vi "Joystick gerakan.vi"() -> ()   [LabVIEW 2019]
uses:
  <vilib>/Platform/TimedLoop/XDataNode/wakeup.ctl
  <vilib>/Platform/TimedLoop/XDataNode/XDNodeRunTimeDep.lvlib
  <vilib>/Platform/TimedLoop/XDataNode/nitl_modes.ctl
  <vilib>/Platform/TimedLoop/XDataNode/timing_clust.ctl
  <vilib>/platform/TimedLoop/XDataNode/XDataNode.xnode
  <vilib>/rvi/interface/nirviReadWriteControl/nirviReadWriteControl.xnode
  <vilib>/rvi/interface/Simulation/niFpgaSimulationCallBeginRW.vi
  <vilib>/rvi/errors/niLvFpgaAdjustHostInterfaceError.vi
  <vilib>/robotics/Steering/Steering Frame/NI_Robotics_Steering Frame.lvclass
  <vilib>/robotics/Steering/Mecanum Steering Frame/NI_Robotics_Mecanum Steering Frame.lvclass
  <vilib>/robotics/Steering/Class Type Definitions/Mecanum Steering Frame.ctl
  <vilib>/robotics/Steering/Class Type Definitions/NI_Robotics_Steering Class Types.lvlib
  <vilib>/robotics/Steering/Mecanum Wheel/Roller Orientation.ctl
  <vilib>/robotics/Steering/Mecanum Wheel/NI_Robotics_Mecanum Wheel.lvclass
  <vilib>/robotics/Steering/Wheel/Rotation Direction.ctl
  <vilib>/robotics/Steering/Wheel/NI_Robotics_Wheel.lvclass
  <vilib>/robotics/Steering/Wheel/Wheel Parameters.ctl
  <vilib>/robotics/Steering/Mecanum Steering Frame/Create Mecanum Steering Frame.vi
  <vilib>/robotics/Steering/Mecanum Wheel/Create Mecanum Wheel.vi
  <vilib>/robotics/Steering/Create Steering Frame/NI_Robotics_Create Steering Frame.xnode
  <vilib>/rvi/interface/nirviCloseFPGA/nirviCloseFPGA.xnode
  <vilib>/rvi/interface/nirviOpenFPGA/nirviOpenFPGA.xnode
  <vilib>/Utility/error.llb/Error Cluster From Error Code.vi
  <vilib>/FPGAPlugInAG/Dynamic/niLvFpga_Close_Dynamic.vi
  Collin's Project/FPGA Bitfiles/MRmecanum_FPGATarget_FPGAMainModified_TerasRobot_LKSN2021.lvbitx
  <vilib>/vision/NI_Vision_Development_Module.lvlib
  NiFpgaLv.dll
  <vilib>/robotics/Steering/Steering Frame/Apply Steering Frame Velocity to Motors.vi
  C:/Program Files (x86)/National Instruments/LabVIEW 2019/vi.lib/robotics/Steering/Special Steering Frame/NI_Robotics_Special Steering Frame.lvclass
  C:/Program Files (x86)/National Instruments/LabVIEW 2019/vi.lib/robotics/Steering/Steering Frame/NI_Robotics_Steering Frame.lvclass
  <vilib>/FPGAPlugInAG/myRIO-1900/niLvFpga_Open_myRIO-1900.vi
  <vilib>/rvi/interface/common/dynamic/niFpgaDynamicAddResources.vi
panel:
  out "Flashlight Number":dbl
  in  "Servo 2":u16=1950
  in  "Max.Servo 2":u16=5000
  in  "Min.Servo 2":u16=1500
  in  "Step Servo 2":u16=50
  out "Kanan Depan":bool
  out "Kanan Belakang":bool
  out "Belakang Kanan":bool
  out "Belakang Kiri":bool
  out "Kiri Belakang":bool
  in  "Stop":bool
  out "Image Out":T1(plugin-control)
  out "Kiri Depan":bool
  out "Depan":bool
  in  "Max.Servo 3":u16=5000
  in  "Min.Servo 3":u16=4400
  in  "Max. Kcp":dbl=500.0
  in  "Min. Kcp":dbl=500.0
  in  "Step Servo 3":u16=50
  in  "Servo 3":u16=5000
  in  "Motor 5":i16=2500
  in  "Putaran":dbl=1700.0
  in  "Kecepatan":dbl=500.0
  # "Maju\nMundur\nKiri\nKanan"
  # "Default Value\n2500"
  # "Putar Kiri\nPutar Kanan"
  # "Std Value : 815"
  # "Std Value : 300\nMin Value : 150\nMax. Value : 400"
  # "Default Value"
  # "Default 3000"
  # "Default 3500"
  # "Default 50"
  # "Servo 3\nDefault Value\n1500"
  # "Default 1000"
  # "Default 2000"
  # "Default 50"
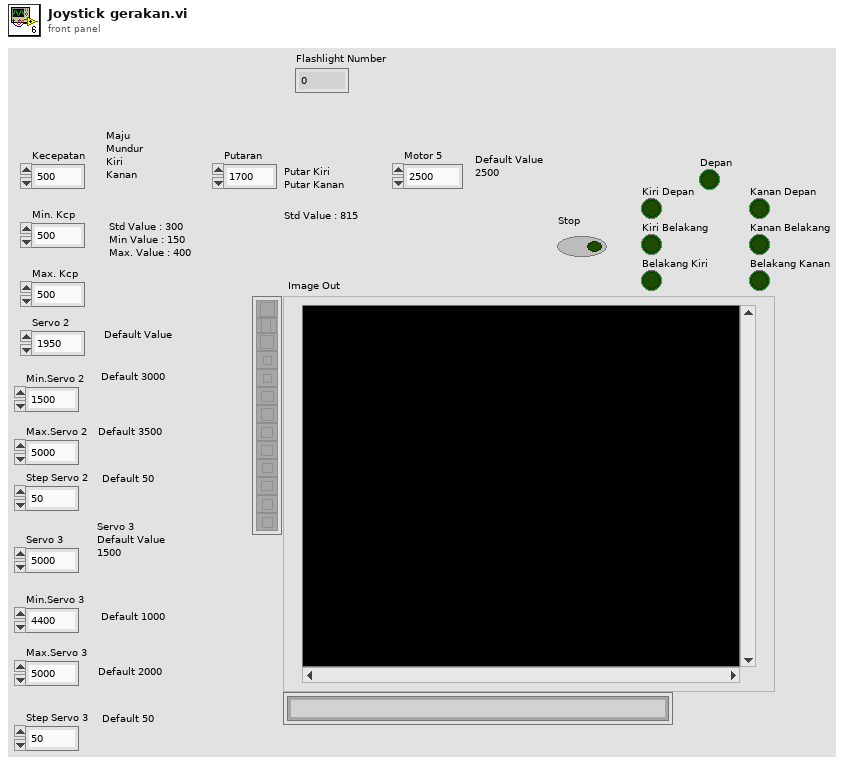
[diagram p1: front panel]
types:
  T1 = typedef "IMAQ Image.ctl" = refnum<image>
  T2 = typedef "NI_Robotics_Steering Class Types.lvlib/Mecanum Steering Frame.ctl" = refnum<class "NI_Robotics_Mecanum Steering Frame.lvclass">
  T3 = typedef "XDNodeRunTimeDep.lvlib/timing_clust.ctl" = cluster{"Expected End [f-1]":u64, "Actual End [f-1]":u64, "Finished Late? [f-1]":bool, "Expected End [i-1]":u64, "Actual End [i-1]":u64, "Finished Late? [i-1]":bool, "Expected Start [i]":u64, "Actual Start [i]":u64, "Expected Start [f]":u64, "Actual Start [f]":u64, "Source Name":string, "Structure Name":string, "Period":i64, "Deadline":i64, "Offset":i64, "Start":i64, "Priority":i32, "Timeout":i32, "Mode":T4, "Wakeup Reason":T5, "Error":errorcluster, "Source Type":string, "Secondary Source Type":string, "Global End Time":u64, "Global Start Time":u64, "Frame Duration":u64, "Iteration Duration":u64, "Assigned CPU":i32, "I/O Scan Engine Mode":u32}
  T4 = typedef "XDNodeRunTimeDep.lvlib/nitl_modes.ctl" = enum32{"No Change", "Process missed periods, maintain original phase", "Discard missed periods, maintain original phase", "Process missed periods, ignore original phase", "Discard missed periods, ignore original phase"}
  T5 = typedef "XDNodeRunTimeDep.lvlib/wakeup.ctl" = enum32{"Normal", "Aborted", "Asynchronous wakeup", "Timing source error", "Timed loop error", "Timeout"}
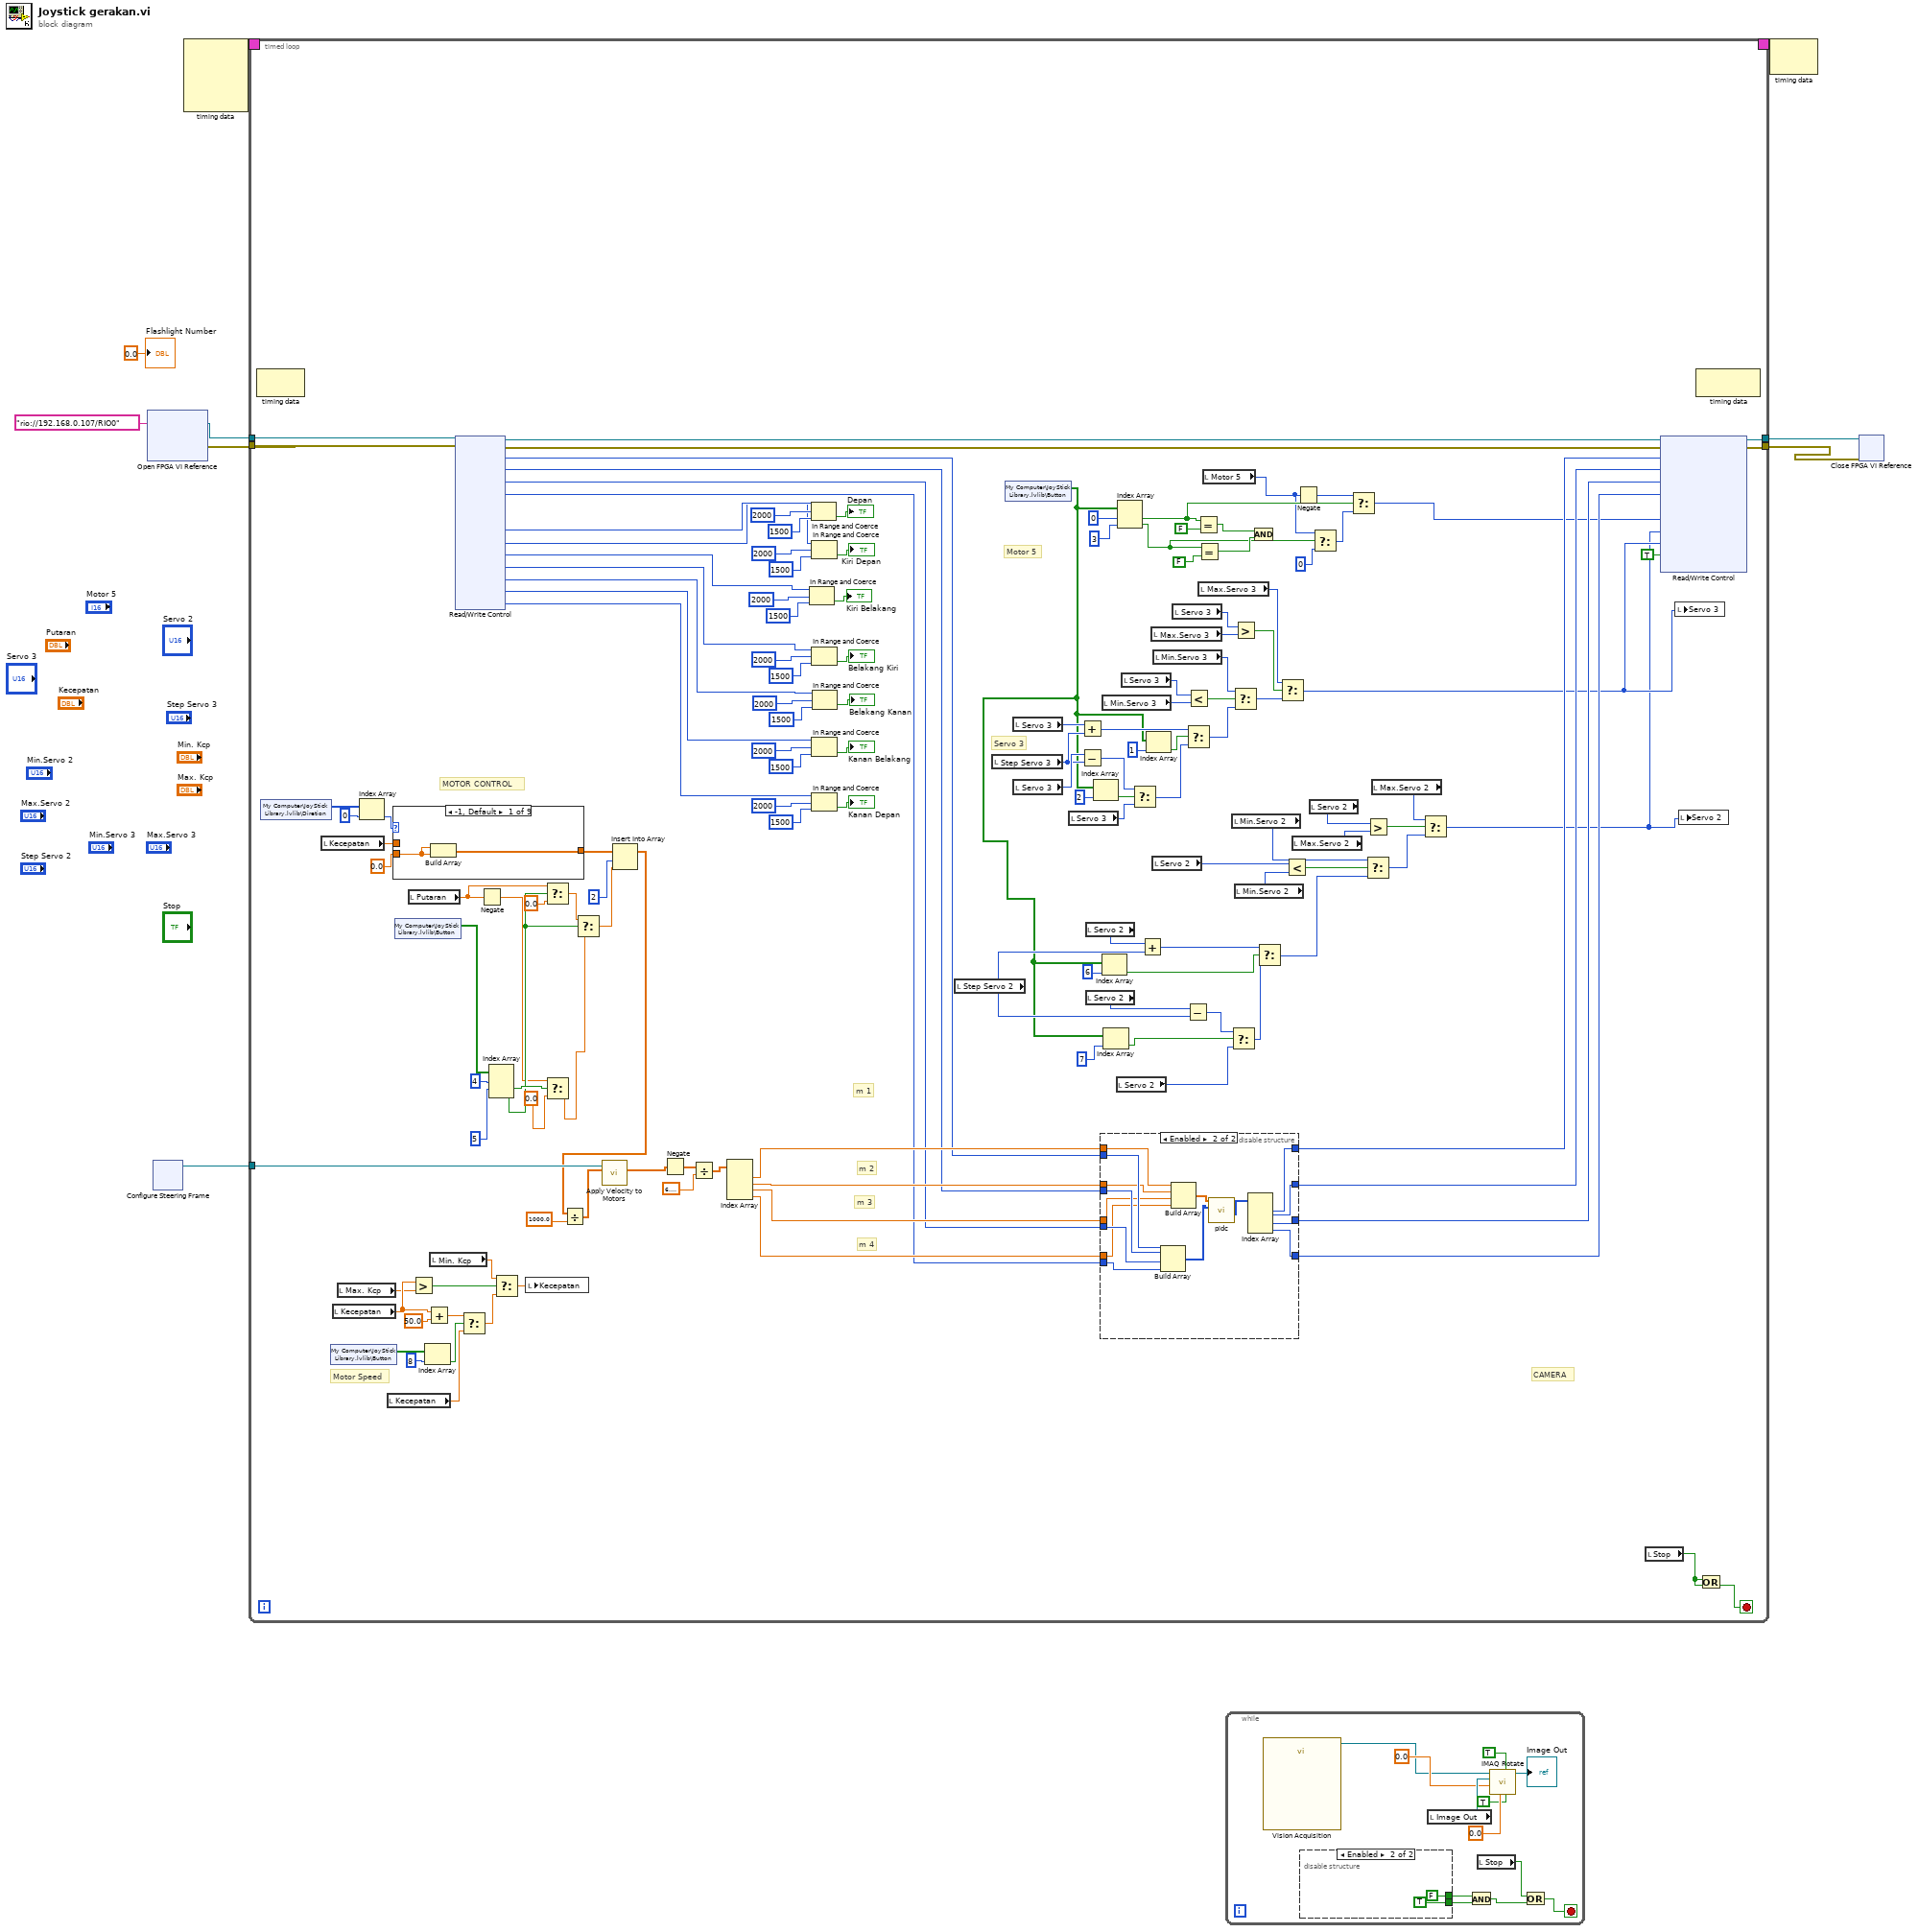
[diagram p0: block diagram]
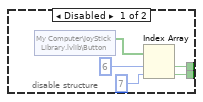
[diagram p2: hidden frame]
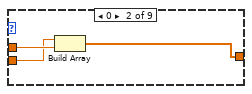
[diagram p3: hidden frame]
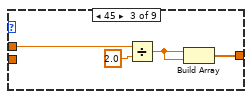
[diagram p4: hidden frame]
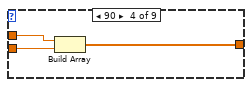
[diagram p5: hidden frame]
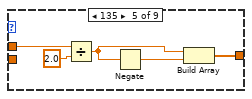
[diagram p6: hidden frame]
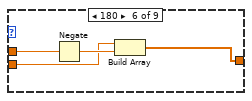
[diagram p7: hidden frame]
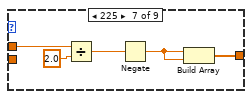
[diagram p8: hidden frame]
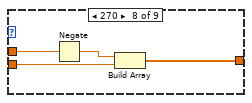
[diagram p9: hidden frame]
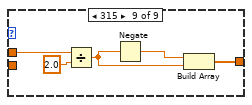
[diagram p10: hidden frame]
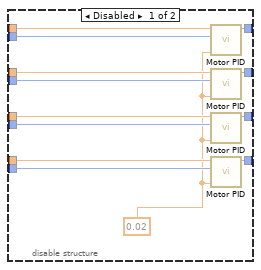
[diagram p11: hidden frame]
diagram:
  n1 = xnode "Open FPGA VI Reference"("resource name"=tag "rio://192.168.0.107/RIO0") -> ("FPGA VI Reference Out"=w4:refnum<k20>, "error out"=w3:errorcluster)  [unwired: 1 in]
  n2 = xnode ("Configure Steering Frame")() -> ("mecanum steering frame out"=w7:T2)  [unwired: 1 in, 1 out]
  n3 = node-c288() -> (w9:T3)  [unwired: 4 in]
  n4 = timed-loop {
    timing: w9 -> [_]
    timing-out: [_] -> w8
    tunnel: w4 -> [w23]
    tunnel: w3 -> [w153]
    tunnel: [w155] -> w6
    tunnel: [w154] -> w5
    tunnel: w7 -> [w152]
    stop <- w71 stop-if-true
    # "CAMERA"
    # "Motor Speed"
    # "Servo 3"
    # "Motor 5"
    # "MOTOR CONTROL"
    # "m 4"
    # "m 3"
    # "m 2"
    # "m 1"
    n5 = node-c288() -> ()  [unwired: 1 in, 1 out]
    n6 = shared-variable "My Computer\\JoyStick Library.lvlib\\Diretion"() -> (w133:i32[])  [unwired: 1 in, 1 out]
    n7 = local read "Kecepatan"() -> (w117:dbl)
    n8 = shared-variable "My Computer\\JoyStick Library.lvlib\\Button"() -> (w100:bool[])  [unwired: 1 in, 1 out]
    n9 = local read "Kecepatan"() -> (w94:dbl)
    n10 = local read "Max. Kcp"() -> (w89:dbl)
    n11 = Index Array(array=w133, index=0) -> (element=w131:i32)
    n12 = local read "Kecepatan"() -> (w91:dbl)
    n13 = case shown="-1, Default" w131 {
      tunnel: [w156 w160 w164 w165 w172 w176 w181 w182 w189] -> w127
      tunnel: w117 -> [_ w159 w162 w167 w170 w175 w180 w185 w186]
      tunnel: 0.0 ("element") -> [w157 w158 _ w166 _ w173 _ w183 _]
      frame -1, Default {
        n14 = Build Array(w157, w157) -> (w156:dbl[])
      }
      frame 0 {
        n15 = Build Array(w158, w159) -> (w160:dbl[])
      }
      frame 45 {
        n16 = Divide(x=w162, y=2.0) -> (x/y=w163:dbl)
        n17 = Build Array(w163, w163) -> (w164:dbl[])
      }
      frame 90 {
        n18 = Build Array(w167, w166) -> (w165:dbl[])
      }
      frame 135 {
        n19 = Divide(x=w170, y=2.0) -> (x/y=w169:dbl)
        n20 = Negate(x=w169) -> (-x=w171:dbl)
        n21 = Build Array(w169, w171) -> (w172:dbl[])
      }
      frame 180 {
        n22 = Negate(x=w175) -> (-x=w174:dbl)
        n23 = Build Array(w173, w174) -> (w176:dbl[])
      }
      frame 225 {
        n24 = Divide(x=w180, y=2.0) -> (x/y=w178:dbl)
        n25 = Negate(x=w178) -> (-x=w179:dbl)
        n26 = Build Array(w179, w179) -> (w181:dbl[])
      }
      frame 270 {
        n27 = Negate(x=w185) -> (-x=w184:dbl)
        n28 = Build Array(w184, w183) -> (w182:dbl[])
      }
      frame 315 {
        n29 = Divide(x=w186, y=2.0 ("Kecepatan")) -> (x/y=w187:dbl)
        n30 = Negate(x=w187) -> (-x=w190:dbl)
        n31 = Build Array(w190, w187) -> (w189:dbl[])
      }
    }
    n32 = shared-variable "My Computer\\JoyStick Library.lvlib\\Button"() -> (w130:bool[])  [unwired: 1 in, 1 out]
    n33 = local read "Putaran"() -> (w115:dbl)
    n34 = Greater?(x=w94, y=w89) -> (0:w98:bool)
    n35 = Index Array(array=w100, index=8) -> (element=w96:bool)
    n36 = Add(x=w94, y=50.0) -> (x+y=w95:dbl)
    n37 = local read "Min. Kcp"() -> (w97:dbl)
    n38 = xnode "Read/Write Control"("FPGA VI Reference In"=w23, "error in"=w153) -> ("FPGA VI Reference Out"=w77:refnum<k20>, "error out"=w72:errorcluster, "ENC M1"=w145:i32, "ENC M2"=w144:i32, "ENC M3"=w143:i32, "ENC M4"=w142:i32, "IR 1"=w76:u16, "IR 3"=w67:u16, "IR 4"=w54:u16, "IR 5"=w53:u16, "IR 6"=w52:u16, "IR 7"=w51:u16, "IR 8"=w47:u16)  [unwired: 2 out]
    n39 = Select(t=w95, s=w96, f=w91) -> (s? t:f=w92:dbl)
    n40 = Negate(x=w115) -> (-x=w114:dbl)
    n41 = Index Array(array=w130, index #1=4 ("index"), index #2=5 ("index")) -> (element #1=w119:bool, element #2=w122:bool)  [unwired: 1 in, 1 out]
    n42 = Select(t=w97, s=w98, f=w92) -> (s? t:f=w90:dbl)
    n43 = local write "Kecepatan"(w90) -> ()
    n44 = Select(t=w115, s=w119, f=0.0) -> (s? t:f=w120:dbl)
    n45 = Select(t=w114, s=w122, f=0.0) -> (s? t:f=w121:dbl)
    n46 = Select(t=w120, s=w119, f=w121) -> (s? t:f=w118:dbl)
    n47 = Insert Into Array(array=w127, index=2, new element=w118) -> (w125:dbl[])
    n48 = Divide(x=w125, y=1000.0) -> (x/y=w136:dbl[])
    n49 = call-poly <vilib>:"Apply Velocity to Motors.vi"("steering frame velocity"=w136, "steering frame in"=w152) -> ("ccw motor velocity setpoints"=w150:dbl[])  [unwired: 5 in, 4 out]
    n50 = Negate(x=w150) -> (-x=w151:dbl[])
    n51 = Divide(x=w151, y=6.283185307179586) -> (x/y=w135:dbl[])
    n52 = Index Array(array=w135) -> (element #1=w149:dbl, element #2=w148:dbl, element #3=w147:dbl, element #4=w146:dbl)  [unwired: 4 in]
    n53 = In Range and Coerce(upper limit=w54, x=u16 2000, lower limit=u16 1500 ("y")) -> (In Range?=→"Kiri Belakang":bool)  [unwired: 1 out]
    n54 = In Range and Coerce(upper limit=w76, x=u16 2000, lower limit=u16 1500 ("y")) -> (In Range?=→"Depan":bool)  [unwired: 1 out]
    n55 = In Range and Coerce(upper limit=w67, x=u16 2000, lower limit=u16 1500 ("y")) -> (In Range?=→"Kiri Depan":bool)  [unwired: 1 out]
    n56 = In Range and Coerce(upper limit=w53, x=u16 2000, lower limit=u16 1500 ("y")) -> (In Range?=→"Belakang Kiri":bool)  [unwired: 1 out]
    n57 = In Range and Coerce(upper limit=w51, x=u16 2000, lower limit=u16 1500 ("y")) -> (In Range?=→"Kanan Belakang":bool)  [unwired: 1 out]
    n58 = In Range and Coerce(upper limit=w47, x=u16 2000, lower limit=u16 1500 ("y")) -> (In Range?=→"Kanan Depan":bool)  [unwired: 1 out]
    n59 = In Range and Coerce(upper limit=w52, x=u16 2000, lower limit=u16 1500 ("y")) -> (In Range?=→"Belakang Kanan":bool)  [unwired: 1 out]
    n60 = local read "Step Servo 2"() -> (w41:u16)
    n61 = local read "Step Servo 3"() -> (w101:u16)
    n62 = shared-variable "My Computer\\JoyStick Library.lvlib\\Button"() -> (w11:bool[])  [unwired: 1 in, 1 out]
    n63 = local read "Servo 3"() -> (w110:u16)
    n64 = local read "Servo 3"() -> (w105:u16)
    n65 = local read "Servo 3"() -> (w103:u16)
    n66 = Add(x=w110, y=w101) -> (x+y=w109:u16)
    n67 = Subtract(x=w105, y=w101) -> (x-y=w107:u16)
    n68 = local read "Servo 2"() -> (w43:u16)
    n69 = local read "Servo 2"() -> (w42:u16)
    n70 = Index Array(array=w11, index=2) -> (element=w108:bool)
    n71 = disable-structure shown="Enabled" {
      disable-tunnel: w149 -> [w203 w211]
      disable-tunnel: w148 -> [w202 w212]
      disable-tunnel: w147 -> [w201 w213]
      disable-tunnel: w146 -> [w200 w214]
      disable-tunnel: w145 -> [w199 w215]
      disable-tunnel: w144 -> [w198 w216]
      disable-tunnel: w143 -> [w197 w217]
      disable-tunnel: w142 -> [w196 w218]
      disable-tunnel: [w195 w208] -> w141
      disable-tunnel: [w194 w204] -> w140
      disable-tunnel: [w193 w207] -> w139
      disable-tunnel: [w192 w206] -> w138
      frame Disabled {
        w191 = 0.02
        n72 = call "Motor PID.vi"("dt[s]"=w191, "encoder"=w199, "vel ref[rps]"=w203) -> ("duty cycle"=w195:i16)  [unwired: 6 in, 2 out]
        n73 = call "Motor PID.vi"("dt[s]"=w191, "encoder"=w198, "vel ref[rps]"=w202) -> ("duty cycle"=w194:i16)  [unwired: 6 in, 2 out]
        n74 = call "Motor PID.vi"("dt[s]"=w191, "encoder"=w197, "vel ref[rps]"=w201) -> ("duty cycle"=w193:i16)  [unwired: 6 in, 2 out]
        n75 = call "Motor PID.vi"("dt[s]"=w191, "encoder"=w196, "vel ref[rps]"=w200) -> ("duty cycle"=w192:i16)  [unwired: 6 in, 2 out]
      }
      frame Enabled {
        n76 = Build Array(w215, w216, w217, w218) -> (w209:i32[])
        n77 = Build Array(w211, w212, w213, w214) -> (w210:dbl[])
        n78 = call "pidc.vi"("input encoder 2"=w209, "input rps"=w210) -> ("Output duty cycle"=w205:i16[])  [unwired: 9 in]
        n79 = Index Array(array=w205) -> (element #1=w208:i16, element #2=w204:i16, element #3=w207:i16, element #4=w206:i16)  [unwired: 4 in]
      }
    }
    n80 = local read "Min.Servo 3"() -> (w82:u16)
    n81 = Index Array(array=w11, index=6) -> (element=w44:bool)
    n82 = Index Array(array=w11, index=7) -> (element=w27:bool)
    n83 = local read "Servo 2"() -> (w30:u16)
    n84 = Index Array(array=w11, index #1=0 ("index"), index #2=3 ("index")) -> (element #1=w18:bool, element #2=w16:bool)
    n85 = local read "Servo 3"() -> (w83:u16)
    n86 = Select(t=w107, s=w108, f=w103) -> (s? t:f=w106:u16)
    n87 = Add(x=w43, y=w41) -> (x+y=w28:u16)
    n88 = Index Array(array=w11, index=1) -> (element=w111:bool)
    n89 = local read "Max.Servo 3"() -> (w87:u16)
    n90 = local read "Servo 2"() -> (w26:u16)
    n91 = local read "Min.Servo 3"() -> (w80:u16)
    n92 = local read "Servo 3"() -> (w88:u16)
    n93 = Subtract(x=w42, y=w41) -> (x-y=w31:u16)
    n94 = Less?(x=w83, y=w82) -> (x < y?=w81:bool)
    n95 = Select(t=w109, s=w111, f=w106) -> (s? t:f=w79:u16)
    n96 = Equal?(x=w18, y=FALSE) -> (x = y?=w20:bool)
    n97 = Equal?(x=w16, y=FALSE) -> (x = y?=w19:bool)
    n98 = local read "Max.Servo 3"() -> (w85:u16)
    n99 = local read "Motor 5"() -> (w15:i16)
    n100 = Select(t=w31, s=w27, f=w30) -> (s? t:f=w29:u16)
    n101 = local read "Min.Servo 2"() -> (w36:u16)
    n102 = Greater?(x=w88, y=w87) -> (0:w86:bool)
    n103 = Select(t=w80, s=w81, f=w79) -> (s? t:f=w78:u16)
    n104 = local read "Min.Servo 2"() -> (w40:u16)
    n105 = And(x=w20, y=w19) -> ()  [unwired: 1 out]
    n106 = Select(t=w28, s=w44, f=w29) -> (s? t:f=w24:u16)
    n107 = Select(t=w85, s=w86, f=w78) -> (s? t:f=w84:u16)
    n108 = Less?(x=w26, y=w40) -> (x < y?=w37:bool)
    n109 = local read "Max.Servo 2"() -> (w38:u16)
    n110 = Negate(x=w15) -> (-x=w17:i16)
    n111 = local read "Servo 2"() -> (w39:u16)
    n112 = Select(t=w15, s=w16, f=i16 0) -> (s? t:f=w13:i16)
    n113 = Select(t=w17, s=w18, f=w13) -> (s? t:f=w12:i16)
    n114 = Select(t=w36, s=w37, f=w24) -> (s? t:f=w34:u16)
    n115 = Greater?(x=w39, y=w38) -> (0:w35:bool)
    n116 = local read "Max.Servo 2"() -> (w33:u16)
    n117 = Select(t=w33, s=w35, f=w34) -> (s? t:f=w32:u16)
    n118 = local read "Stop"() -> (w25:bool)
    n119 = xnode "Read/Write Control"("FPGA VI Reference In"=w77, "error in"=w72, "M1"=w141, "M2"=w140, "M3"=w139, "M4"=w138, "M5"=w12, "SERVO 2"=w32, "SERVO 3"=w84, "DIO.A_13.VAL"=TRUE) -> ("FPGA VI Reference Out"=w155:refnum<k20>, "error out"=w154:errorcluster)  [unwired: 2 in]
    n120 = local write "Servo 3"(w84) -> ()
    n121 = local write "Servo 2"(w32) -> ()
    n122 = node-c288() -> ()  [unwired: 1 in, 1 out]
    n123 = Or(x=w25, y=w25) -> (x .or. y?=w71:bool)
  }
  n124 = while {
    stop <- w225 stop-if-true
    n125 = call "Vision Acquisition"() -> ("Image Out"=w229:T1)  [unwired: 25 in, 2 out]
    n126 = disable-structure shown="Enabled" {
      disable-tunnel: [w234 FALSE ("Boolean")] -> w227
      disable-tunnel: [w233 TRUE ("Boolean")] -> w226
      frame Disabled {
        n127 = shared-variable "My Computer\\JoyStick Library.lvlib\\Button"() -> (w237:bool[])  [unwired: 1 in, 1 out]
        n128 = Index Array(array=w237, index #1=6 ("index"), index #2=7 ("index")) -> (element #1=w234:bool, element #2=w233:bool)
      }
      frame Enabled {
      }
    }
    n129 = local read "Image Out"() -> (w232:T1)
    n130 = And(x=w227, y=w226) -> (x .and. y?=w224:bool)
    n131 = local read "Stop"() -> (w223:bool)
    n132 = call "IMAQ Rotate"("Use Bilinear Interpolation"=TRUE, "Maintain Size"=TRUE, "Replace Value"=sgl 0.0, "Angle (degrees)"=sgl 0.0, "Image Dst"=w232, "Image Src"=w229) -> ("Image Dst Out"=→"Image Out":T1)  [unwired: 4 in, 1 out]
    n133 = Or(x=w223, y=w224) -> (x .or. y?=w225:bool)
  }
  n134 = node-c288(w8) -> ()  [unwired: 1 out]
  n135 = xnode "Close FPGA VI Reference"("FPGA VI Reference In"=w6, "error in"=w5) -> ()  [unwired: 1 out]
  "Flashlight Number" <- 0.0 ("Flashlight Number")
